vi "FindEventRefnumRecursive.vi"(7 "count in":i32, 8 "InNamedTypedef?":bool, 9 "Event name":string, 10 "Event holder typedef":string, 11 "Data Type":variant) -> (2 "Found?":bool, 5 "count out":i32)   [LabVIEW 2024, in "AddNewEvent.lvlib"]
uses:
  AddNewEvent.lvlib
  <vilib>/Utility/Data Type/NI_Data Type.lvlib
panel:
  out "Data Type 2":variant
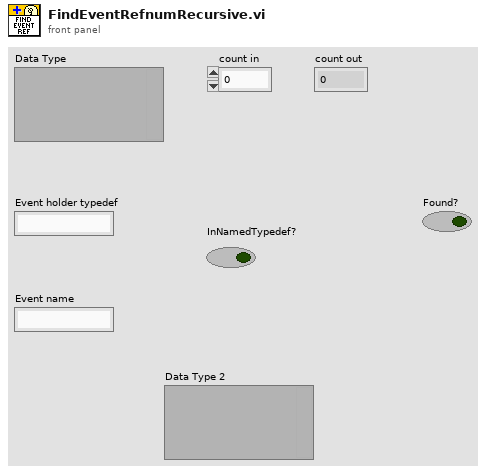
[diagram p1: front panel]
types:
  T1 = typedef "NI_Data Type.lvlib/Data Type.ctl" = enum8{"Invalid Type", "Void", "I8", "I16", "I32", "I64", "U8", "U16", "U32", "U64", "Single Float", "Double Float", "Extended Float", "Single Complex", "Double Complex", "Extended Complex", "Enum U8", "Enum U16", "Enum U32", "Enum U64", "Single Float With Unit", "Double Float With Unit", "Extended Float With Unit", "Single Complex with Unit", "Double Complex with Unit", "Extended Complex with Unit", "Boolean", "String", "Path", "Picture", "Tag", "Array", "Cluster", "Variant", "LV Variant", "Waveform", "Timestamp", "Digital Waveform", "Digital Data", "ExpressData", "Refnum", "External Data", "VI", "Poly VI", "LabVIEW Class Instance", "Fixed Point", "Set Collection", "Map Collection"}
  T2 = typedef "NI_Data Type.lvlib/Type Definition Info.ctl" = cluster{"Name":string, "Timestamp":u32}
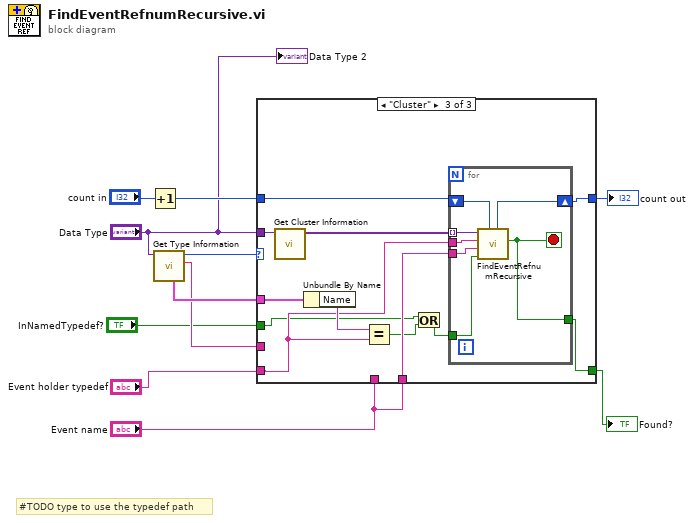
[diagram p0: block diagram]
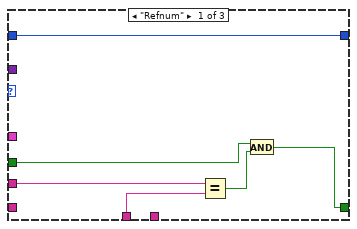
[diagram p2: hidden frame]
diagram:
  # "#TODO type to use the typedef path"
  n1 = Increment(x="count in") -> (x+1=w11:i32)
  n2 = call <vilib>:"Get Type Information.vi"("variant"="Data Type") -> ("name"=w3:string, "type"=w8:T1, "type definition info"=w6:T2)  [unwired: 6 in, 2 out]
  n3 = case shown="\"Cluster\"" w8 {
    tunnel: "Data Type" -> [_ _ w30]
    tunnel: w11 -> [w17 w18 w28]
    tunnel: [w17 w18 w27] -> w9
    tunnel: "Event name" -> [_ _ w26]
    tunnel: w6 -> [_ _ w25]
    tunnel: "Event holder typedef" -> [_ _ w23]
    tunnel: "Event name" -> [w16 _ _]
    tunnel: w3 -> [w15 _ _]
    tunnel: [w12 _ w19] -> w2
    tunnel: "InNamedTypedef?" -> [w14 _ w21]
    frame "Refnum" {
      n4 = Equal?(x=w15, y=w16) -> (x = y?=w13:bool)
      n5 = And(x=w14, y=w13) -> (x .and. y?=w12:bool)
    }
    frame Default {
    }
    frame "Cluster" {
      n6 = call <vilib>:"Get Cluster Information.vi"("variant"=w30) -> ("cluster elements"=w29:variant[])  [unwired: 9 in, 1 out]
      n7 = Unbundle By Name(w25) -> ("Name"=w24:string)
      n8 = Equal?(x=w24, y=w23) -> (x = y?=w22:bool)
      n9 = Or(x=w21, y=w22) -> (x .or. y?=w20:bool)
      n10 = for {
        tunnel: w29 -> [w37] mode=indexing
        shift-right: [w36] -> w27
        shift-left: w28 -> [w35]
        tunnel: w26 -> [w33]
        tunnel: w20 -> [w34]
        tunnel: w23 -> [w32]
        tunnel: [w31] -> w19
        stop <- w31 stop-if-true
        n11 = call "FindEventRefnumRecursive.vi"("count in"=w35, "InNamedTypedef?"=w34, "Event name"=w33, "Event holder typedef"=w32, "Data Type"=w37) -> ("Found?"=w31:bool, "count out"=w36:i32)  [unwired: 5 in]
      }
    }
  }
  "Found?" <- w2
  "count out" <- w9
  "Data Type 2" <- "Data Type"
